vi "Teleop.vi"(10 "Match Info":T1={"Autonomous Elapsed Seconds"=0.0, "TeleOp Elapsed Seconds"=0.0, "Disabled Elapsed Seconds"=0.0, "Visited Autonomous"=FALSE, "Visited TeleOp"=FALSE, "Visited Disabled"=FALSE, "Autonomous Settings"={"Autonomous Style"=enum."Independent", "VI Refnum"=refnum}}, 11 "Call Context":T2) -> ()   [LabVIEW 2014]
doc: "This VI is called for each TeleOp packet received from the DS where the robot is not disabled. It is often used to read from the joysticks and update I/O or to update setpoints for timed control loops. It should complete and return within 20 milliseconds or it may miss DS packets."
uses:
  <vilib>/Rock Robotics/WPI/DriverStation/WPI_DriverStationDerivedRobotMode.ctl
  <vilib>/Rock Robotics/WPI/DriverStation/WPI_DriverStationMatch Info.ctl
  <vilib>/Rock Robotics/WPI/RobotDrive/WPI_RobotDriveGetSetRefNum.vi
  <vilib>/Rock Robotics/WPI/Joystick/WPI_JoystickGetSetRefNum.vi
  <vilib>/Rock Robotics/Network Tables/SD Read Boolean.vi
  <vilib>/Rock Robotics/Network Tables/SD Read Number.vi
  Robot Global Data.vi
  <vilib>/Rock Robotics/Network Tables/SD Write Numeric Array.vi
  <vilib>/Rock Robotics/Network Tables/SD Write Boolean Array.vi
panel:
  out "Sample Slider 0":dbl(slide) scale=0.0..5.0
  out "Sample Boolean 1":bool
  out "Sample Boolean 0":bool
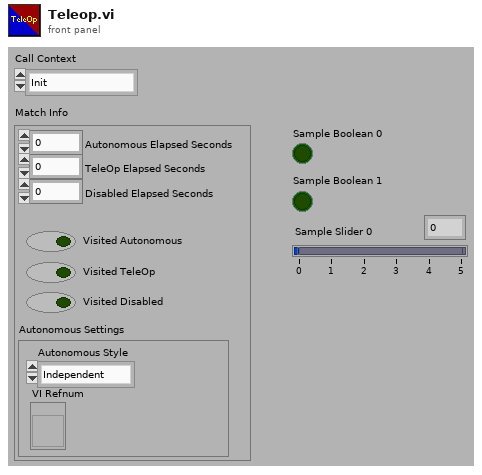
[diagram p1: front panel]
types:
  T1 = typedef "WPI_DriverStationMatch Info.ctl" = cluster{"Autonomous Elapsed Seconds":dbl, "TeleOp Elapsed Seconds":dbl, "Disabled Elapsed Seconds":dbl, "Visited Autonomous":bool, "Visited TeleOp":bool, "Visited Disabled":bool, "Autonomous Settings":cluster{"Autonomous Style":enum16{"Iterative", "Independent"}, "VI Refnum":refnum<vi>}}
  T2 = typedef "WPI_DriverStationDerivedRobotMode.ctl" = enum16{"Init", "Execute", "Stop"}
  T3 = typedef "WPI_JoystickDevRef.ctl" = cluster{"Device":T4}
  T4 = typedef "WPI_JoystickDeviceEnum.ctl" = enum16{"USB 0", "USB 1", "USB 2", "USB 3", "USB 4", "USB 5"}
  T5 = typedef "WPI_RobotDriveDevRef.ctl" = cluster{"DevStatus":errorcluster, "Motors[]":T6[], "Square Inputs":bool, "Max Output":dbl}
  T6 = typedef "WPI_MotorControlDeviceRef.ctl" = cluster{"DeviceStatus":errorcluster, "Type":T7, "PWM":cluster{"Controller":T8, "PWM Channel":T9, "DeadBand":T10}, "CAN":cluster{"Device Number":u8, "Control Mode":T11, "Semaphore":T12, "Max Vout":dbl, "TalonSRX Control Mode":T13}, "Invert":bool, "TransformRef":T14, "InvTransformRef":T14}
  T7 = typedef "WPI_MotorControlType.ctl" = enum16{"PWM", "CAN", "CANTalonSRX"}
  T8 = typedef "FPGA_TypedefDigitalModule.ctl" = enum16{"Controller 1"}
  T9 = typedef "FPGA_DIOPWMChannel.ctl" = enum8{"PWM 0", "PWM 1", "PWM 2", "PWM 3", "PWM 4", "PWM 5", "PWM 6", "PWM 7", "PWM 8", "PWM 9", "PWM MXP 0", "PWM MXP 1", "PWM MXP 2", "PWM MXP 3", "PWM MXP 4", "PWM MXP 5", "PWM MXP 6", "PWM MXP 7", "PWM MXP 8", "PWM MXP 9", "Invalid"}
  T10 = typedef "WPI_PWMDeadband.ctl" = cluster{"Name":string, "maxPositivePwm":i32, "minPositivePwm":i32, "centerPwm":i32, "maxNegativePwm":i32, "minNegativePwm":i32, "angularRange":u16}
  T11 = typedef "WPI_CANJaguar_ControlMode.ctl" = enum8{"Percent VBus", "Current", "Speed", "Position", "Voltage"}
  T12 = typedef "Semaphore RefNum" = refnum<k1>
  T13 = typedef "WPI_CANTalonSRX_APIControlMode.ctl" = enum8{"Percent VBus", "Speed", "Position", "Slave", "Unchanged / Invalid"}
  T14 = typedef "WPI_PWMTransform_ConPane.ctl" = refnum<vi>
  T15 = typedef "WPI_DigitalInputDevRef.ctl" = cluster{"DevStatus":errorcluster, "DIO Channel":T16, "Controller":T8}
  T16 = typedef "FPGA_DIOChannel.ctl" = enum8{"DIO 0", "DIO 1", "DIO 2", "DIO 3", "DIO 4", "DIO 5", "DIO 6", "DIO 7", "DIO 8", "DIO 9", "DIO MXP 0", "DIO MXP 1", "DIO MXP 2", "DIO MXP 3", "DIO MXP 4", "DIO MXP 5", "DIO MXP 6", "DIO MXP 7", "DIO MXP 8", "DIO MXP 9", "DIO MXP 10", "DIO MXP 11", "DIO MXP 12", "DIO MXP 13", "DIO MXP 14", "DIO MXP 15", "Invalid"}
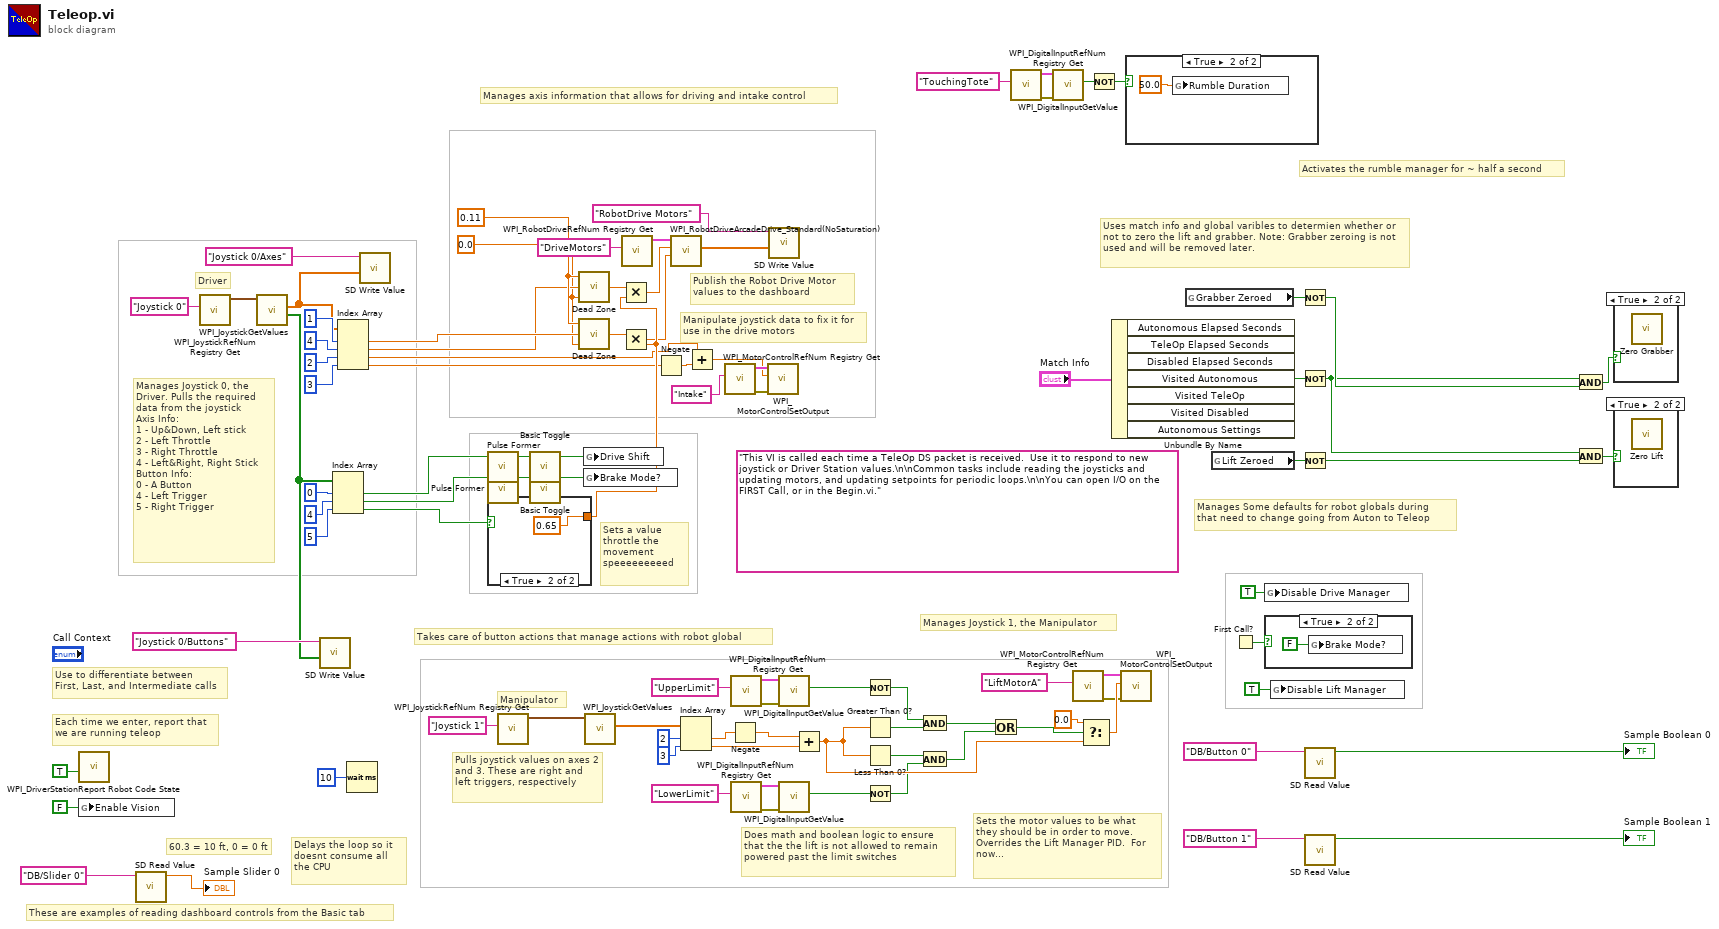
[diagram p0: block diagram]
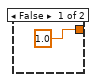
[diagram p4: hidden frame]
diagram:
  w74 = 0.11 ("Range")
  w46 = 0.0
  (unwired) "This VI is called each time a TeleOp DS packet is received.  Use it to respond to new joystick or Driver Station values.\n\nCommon tasks include reading the joysticks and updating motors, and updating setpoints for periodic loops.\n\nYou can open I/O on the FIRST Call, or in the Begin.vi."
  # "Activates the rumble manager for ~ half a second"
  # "Manipulate joystick data to fix it for use in the drive motors"
  # "Delays the loop so it doesnt consume all the CPU"
  # "Manages axis information that allows for driving and intake control"
  # "Sets a value throttle the movement speeeeeeeeed"
  # "Takes care of button actions that manage actions with robot global"
  # "Manages Joystick 0, the Driver. Pulls the required data from the joystick\nAxis Info:\n1 - Up&Down, Left stick\n2 - Left Throttle\n3 - Right Throttle\n4 - Left&Right, Right Stick\nButton Info:\n0 - A Button \n4 - Left Trigger\n5 - Right Trigger"
  # "Sets the motor values to be what they should be in order to move. Overrides the Lift Manager PID.  For now..."
  # "Does math and boolean logic to ensure that the the lift is not allowed to remain powered past the limit switches"
  # "Pulls joystick values on axes 2 and 3. These are right and left triggers, respectively"
  # "Manages Joystick 1, the Manipulator"
  # "Manages Some defaults for robot globals during\nthat need to change going from Auton to Teleop"
  # "Uses match info and global varibles to determien whether or not to zero the lift and grabber. Note: Grabber zeroing is not used and will be removed later."
  # "60.3 = 10 ft, 0 = 0 ft"
  # "Manipulator"
  # "Driver"
  # "These are examples of reading dashboard controls from the Basic tab"
  # "Publish the Robot Drive Motor\nvalues to the dashboard"
  # "Each time we enter, report that\nwe are running teleop"
  # "Use to differentiate between\nFirst, Last, and Intermediate calls"
  n1 = call <vilib>:"WPI_DriverStationReport Robot Code State.vi"("TeleOp"=TRUE ("Autonomous")) -> ()  [unwired: 10 in, 1 out]
  n2 = global write "Robot Global Data.vi" "Enable Vision"(FALSE ("Enable Vision")) -> ()
  n3 = call-poly <vilib>:"SD Read Value.vi"("Name"="DB/Slider 0" ("refnum name")) -> ("Numeric"=→"Sample Slider 0":dbl)  [unwired: 8 in, 2 out]
  n4 = call <vilib>:"WPI_JoystickRefNum Registry Get.vi"("refnum name"="Joystick 0") -> ("JoystickDevRef"=w72:T3)  [unwired: 1 in, 9 out]
  n5 = call <vilib>:"WPI_JoystickGetValues.vi"("JoystickDevRef"=w72) -> ("Buttons"=w6:bool[], "Axes"=w69:dbl[])  [unwired: 6 in, 3 out]
  n6 = call-poly <vilib>:"SD Write Value.vi"("Boolean Array"=w6, "Name"="Joystick 0/Buttons") -> ()  [unwired: 8 in, 2 out]
  n7 = Index Array(array=w6, index #1=0 ("index"), index #2=4 ("index"), index #3=5 ("index")) -> (element #1=w66:bool, element #2=w54:bool, element #3=w48:bool)
  n8 = Index Array(array=w69, index #1=1 ("index"), index #2=4 ("index"), index #3=2 ("index"), index #4=3 ("index")) -> (element #1=w68:dbl, element #2=w67:dbl, element #3=w38:dbl, element #4=w39:dbl)
  n9 = Wait (ms)(milliseconds to wait=u32 10) -> ()  [unwired: 1 out]
  n10 = call-poly <vilib>:"SD Write Value.vi"("Numeric Array"=w69, "Name"="Joystick 0/Axes") -> ()  [unwired: 8 in, 2 out]
  n11 = call "Pulse Former.vi"("Input"=w66) -> ("Pulse"=w78:bool)  [unwired: 4 in]
  n12 = call "Pulse Former.vi"("Input"=w54) -> ("Pulse"=w52:bool)  [unwired: 4 in]
  n13 = case shown="True" w48 {
    tunnel: [1.0 0.65] -> w49
    frame False {
    }
    frame True {
    }
  }
  n14 = call <vilib>:"WPI_JoystickRefNum Registry Get.vi"("refnum name"="Joystick 1") -> ("JoystickDevRef"=w92:T3)  [unwired: 1 in, 9 out]
  n15 = call "Basic Toggle.vi"("Input"=w78) -> ("Output"=w77:bool)  [unwired: 4 in]
  n16 = call "Basic Toggle.vi"("Input"=w52) -> ("Output"=w45:bool)  [unwired: 4 in]
  n17 = call "Dead Zone.vi"("Dead Value"=w46, "Data"=w67, "Range"=w74) -> ("Dead Zoned Data"=w51:dbl)
  n18 = call "Dead Zone.vi"("Dead Value"=w46, "Data"=w68, "Range"=w74) -> ("Dead Zoned Data"=w50:dbl)
  n19 = global write "Robot Global Data.vi" "Drive Shift"(w77) -> ()
  n20 = global write "Robot Global Data.vi" "Brake Mode?"(w45) -> ()
  n21 = call <vilib>:"WPI_JoystickGetValues.vi"("JoystickDevRef"=w92) -> ("Axes"=w81:dbl[])  [unwired: 6 in, 4 out]
  n22 = Multiply(x=w51, y=w49) -> (x*y=w44:dbl)
  n23 = Multiply(x=w50, y=w49) -> (x*y=w43:dbl)
  n24 = call <vilib>:"WPI_RobotDriveRefNum Registry Get.vi"("refnum name"="DriveMotors") -> ("RobotDriveDevRef"=w53:T5)  [unwired: 1 in, 9 out]
  n25 = Negate(x=w39) -> (-x=w37:dbl)
  n26 = call <vilib>:"WPI_RobotDriveArcadeDrive_Standard(NoSaturation).vi"("Y axis value"=w43, "X axis value"=w44, "RobotDriveDevRef"=w53) -> ("Motor Values"=w83:dbl[])  [unwired: 1 in, 7 out]
  n27 = Index Array(array=w81, index #1=2 ("index"), index #2=3 ("index")) -> (element #1=w8:dbl, element #2=w7:dbl)
  n28 = Add(x=w38, y=w37) -> (x+y=w32:dbl)
  n29 = call <vilib>:"WPI_MotorControlRefNum Registry Get.vi"("refnum name"="Intake") -> ("error out"=w34:errorcluster, "MotorControlDevRef"=w33:T6)  [unwired: 9 in]
  n30 = Negate(x=w8) -> (-x=w30:dbl)
  n31 = call <vilib>:"WPI_DigitalInputRefNum Registry Get.vi"("refnum name"="UpperLimit") -> ("error out"=w20:errorcluster, "DigitalInputDevRef"=w21:T15)  [unwired: 9 in]
  n32 = call <vilib>:"WPI_DigitalInputRefNum Registry Get.vi"("refnum name"="LowerLimit") -> ("error out"=w22:errorcluster, "DigitalInputDevRef"=w23:T15)  [unwired: 9 in]
  n33 = call <vilib>:"WPI_MotorControlSetOutput.vi"("error in (no error)"=w34, "Output"=w32, "MotorControlDevRef"=w33) -> ()  [unwired: 6 in, 3 out]
  n34 = call-poly <vilib>:"SD Write Value.vi"("Numeric Array"=w83, "Name"="RobotDrive Motors") -> ()  [unwired: 8 in, 2 out]
  n35 = call <vilib>:"WPI_DigitalInputGetValue.vi"("error in (no error)"=w20, "DigitalInputDevRef"=w21) -> ("Value"=w26:bool)  [unwired: 7 in, 2 out]
  n36 = call <vilib>:"WPI_DigitalInputGetValue.vi"("error in (no error)"=w22, "DigitalInputDevRef"=w23) -> ("Value"=w27:bool)  [unwired: 7 in, 2 out]
  n37 = Add(x=w30, y=w7) -> (x+y=w29:dbl)
  n38 = Not(x=w26) -> (.not. x?=w17:bool)
  n39 = Greater Than 0?(x=w29) -> (x > 0?=w14:bool)
  n40 = Less Than 0?(x=w29) -> (x < 0?=w15:bool)
  n41 = Not(x=w27) -> (.not. x?=w16:bool)
  n42 = And(x=w17, y=w14) -> (x .and. y?=w18:bool)
  n43 = And(x=w15, y=w16) -> (x .and. y?=w19:bool)
  n44 = Or(x=w18, y=w19) -> (x .or. y?=w12:bool)
  n45 = call <vilib>:"WPI_DigitalInputRefNum Registry Get.vi"("refnum name"="TouchingTote") -> ("error out"=w4:errorcluster, "DigitalInputDevRef"=w3:T15)  [unwired: 9 in]
  n46 = call <vilib>:"WPI_DigitalInputGetValue.vi"("error in (no error)"=w4, "DigitalInputDevRef"=w3) -> ("Value"=w2:bool)  [unwired: 7 in, 2 out]
  n47 = call <vilib>:"WPI_MotorControlRefNum Registry Get.vi"("refnum name"="LiftMotorA") -> ("error out"=w10:errorcluster, "MotorControlDevRef"=w11:T6)  [unwired: 9 in]
  n48 = Select(t=0.0, s=w12, f=w29) -> (s? t:f=w28:dbl)
  n49 = Not(x=w2) -> (.not. x?=w1:bool)
  n50 = Unbundle By Name("Match Info") -> ("Visited Autonomous"=w63:bool)  [unwired: 6 out]
  n51 = call <vilib>:"WPI_MotorControlSetOutput.vi"("error in (no error)"=w10, "Output"=w28, "MotorControlDevRef"=w11) -> ()  [unwired: 6 in, 3 out]
  n52 = case shown="True" w1 {
    frame False {
    }
    frame True {
      n53 = global write "Robot Global Data.vi" "Rumble Duration"(50.0) -> ()
    }
  }
  n54 = global read "Robot Global Data.vi" "Grabber Zeroed"() -> (w61:bool)
  n55 = global read "Robot Global Data.vi" "Lift Zeroed"() -> (w57:bool)
  n56 = First Call?() -> (First Call?: T/F=w35:bool)
  n57 = global write "Robot Global Data.vi" "Disable Drive Manager"(TRUE ("Disable Drive Manager")) -> ()
  n58 = case shown="True" w35 {
    frame False {
    }
    frame True {
      n59 = global write "Robot Global Data.vi" "Brake Mode?"(FALSE) -> ()
    }
  }
  n60 = global write "Robot Global Data.vi" "Disable Lift Manager"(TRUE) -> ()
  n61 = Not(x=w61) -> (.not. x?=w62:bool)
  n62 = Not(x=w63) -> (.not. x?=w59:bool)
  n63 = Not(x=w57) -> (.not. x?=w58:bool)
  n64 = call-poly <vilib>:"SD Read Value.vi"("Name"="DB/Button 0" ("refnum name")) -> ("Boolean"=→"Sample Boolean 0":bool)  [unwired: 8 in, 2 out]
  n65 = call-poly <vilib>:"SD Read Value.vi"("Name"="DB/Button 1" ("refnum name")) -> ("Boolean"=→"Sample Boolean 1":bool)  [unwired: 8 in, 2 out]
  n66 = And(x=w59, y=w62) -> (x .and. y?=w64:bool)
  n67 = And(x=w59, y=w58) -> (x .and. y?=w60:bool)
  n68 = case shown="True" w64 {
    frame False {
    }
    frame True {
      n69 = call "Zero Grabber.vi"() -> ()  [unwired: 11 in, 1 out]
    }
  }
  n70 = case shown="True" w60 {
    frame False {
    }
    frame True {
      n71 = call "Zero Lift.vi"() -> ()  [unwired: 11 in, 1 out]
    }
  }
